vi "BCU参数读取-Auto.vi"(8 "CAN端口":u16(ring), 9 "设备索引号":u16(ring), 10 "CAN卡类型":u32(ring)=21, 11 "Myindex":dbl=1.0) -> (3 "成功":bool)   [LabVIEW 2013] (continued)
                            n1192 = local read "CAN端口"() -> (w1917:u16)
                            n1193 = local write "命令序号"(w1922) -> ()
                            n1194 = stacked-sequence {
                              tunnel: w1923 -> [_ w1931]
                              tunnel: w1922 -> [_ w1930]
                              tunnel: w1921 -> [_ w1929]
                              tunnel: w1920 -> [_ w1928]
                              tunnel: w1919 -> [_ w1927]
                              tunnel: w1918 -> [_ w1926]
                              tunnel: w1917 -> [_ w1925]
                              frame #0 {
                              }
                              frame #1 {
                                n1195 = control-ref of="流控帧"() -> (w1924:refnum<vi>)
                                n1196 = call "多帧发送机制(EV05).vi"("can卡类型"=w1927, "设备索引号"=w1926, "CAN端口"=w1925, "命令"=w1931, "板号"=w1929, "命令序号"=w1930, "输入数据"=w1928, "流控帧"=w1924) -> ()  [unwired: 1 in, 11 out]
                              }
                            }
                          }
                          frame #4 {
                            n1197 = while {
                              tunnel: [w1936] -> w1933
                              tunnel: [w1934] -> w1932
                              i -> [w1939]
                              stop <- w1936 stop-if-true
                              n1198 = local read "强制终止读写标记"() -> (w1935:bool)
                              n1199 = local read "写入超时"() -> (w1934:bool)
                              n1200 = Greater Or Equal?(x=w1939, y=20) -> (x >= y?=w1937:bool)
                              n1201 = Compound Arithmetic op=OR(w1935, w1934, w1937) -> (w1936:bool)
                              n1202 = Wait Until Next ms Multiple(millisecond multiple=u32 100 ("毫秒倍数")) -> ()  [unwired: 1 out]
                            }
                          }
                          frame #5 {
                            n1203 = case shown="假" w1948 {
                              tunnel: w1947 -> [w1959 _]
                              tunnel: [w1954 w1971] -> w1946
                              tunnel: w1945 -> [w1953 _]
                              tunnel: w1944 -> [w1952 w1971]
                              tunnel: [w1951 w1970] -> w1941
                              tunnel: w1943 -> [w1950 _]
                              tunnel: w1942 -> [w1949 w1970]
                              frame False {
                                n1204 = local read "重试次数"() -> (w1958:u8)
                                n1205 = Increment(x=w1958) -> (x+1=w1957:u8)
                                n1206 = local write "重试次数"(w1957) -> ()
                                n1207 = Greater Or Equal?(x=w1957, y=u8 4) -> (x >= y?=w1956:bool)
                                n1208 = case shown="真" w1956 {
                                tunnel: w1959 -> [_ w1964]
                                tunnel: [w1961 w1963] -> w1954
                                tunnel: w1953 -> [w1961 _]
                                tunnel: w1952 -> [_ w1963]
                                tunnel: [w1960 w1962] -> w1951
                                tunnel: w1950 -> [w1960 _]
                                tunnel: w1949 -> [_ w1962]
                                frame False {
                                }
                                frame True {
                                n1209 = control-ref of="结果"() -> (w1966:refnum<vi>)
                                n1210 = Concatenate Strings(w1964, "     读取失败" ("字符串")) -> (w1968:string)
                                n1211 = Build Array(w1968) -> (w1965:string[])
                                n1212 = call "表格编辑.vi"("新元素/子数组"=w1965, "活动单元格:单元格背景色"=u32 16740749, "MCListbox引用句柄"=w1966) -> ()  [unwired: 9 out]
                                }
                                }
                              }
                              frame True {
                              }
                            }
                          }
                          frame #6 {
                            n1213 = And(x=w1973, y=w1975) -> (x .and. y?=w1974:bool)
                            n1214 = case shown="真" w1974 {
                              frame False {
                              }
                              frame True {
                                n1215 = local write "强制终止读写标记"(FALSE ("强制停止")) -> ()
                                n1216 = control-ref of="结果"() -> (w1978:refnum<vi>)
                                n1217 = Concatenate Strings("读取完成" ("字符串")) -> (w1980:string)
                                n1218 = Build Array(w1980) -> (w1977:string[])
                                n1219 = call "表格编辑.vi"("新元素/子数组"=w1977, "活动单元格:单元格背景色"=u32 21937, "MCListbox引用句柄"=w1978) -> ()  [unwired: 9 out]
                              }
                            }
                            n1220 = Wait (ms)(milliseconds to wait=u32 100 ("等待时间（毫秒）")) -> ()  [unwired: 1 out]
                          }
                        }
                      }
                    }
                  }
                  n1221 = local read "强制终止读写标记"() -> (w1745:bool)
                  n1222 = Or(x=w1745, y=w1744) -> (x .or. y?=w1742:bool)
                }
              }
            }
            frame #3 {
              n1223 = case shown="假" FALSE {
                tunnel: w2072 -> [w2073 _]
                frame False {
                  n1224 = case shown="\"主板\", 默认" w2073 {
                    frame "主板", Default {
                      w2074 = "BCURESULT" ("section")
                      n1225 = global read "读配置文件全局.vi" "电池额定实际容量判定"() -> (w2096:bool)
                      n1226 = global read "读配置文件全局.vi" "电池充放电次数判定"() -> (w2085:bool)
                      n1227 = global read "读配置文件全局.vi" "加热控制参数判定"() -> (w2083:bool)
                      n1228 = global read "读配置文件全局.vi" "配置文件版本判定"() -> (w2095:bool)
                      n1229 = global read "读配置文件全局.vi" "充电控制参数判定"() -> (w2089:bool)
                      n1230 = global read "读配置文件全局.vi" "通道电压数判定"() -> (w2101:bool)
                      n1231 = global read "读配置文件全局.vi" "电压起始值判定"() -> (w2100:bool)
                      n1232 = global read "读配置文件全局.vi" "温度起始值判定"() -> (w2098:bool)
                      n1233 = global read "读配置文件全局.vi" "充放电安时判定"() -> (w2087:bool)
                      n1234 = global read "读配置文件全局.vi" "电池包组号判定"() -> (w2086:bool)
                      n1235 = global read "读配置文件全局.vi" "电池信息1判定"() -> (w2088:bool)
                      n1236 = global read "读配置文件全局.vi" "从板个数判定"() -> (w2104:bool)
                      n1237 = global read "读配置文件全局.vi" "产品编号判定"() -> (w2103:bool)
                      n1238 = global read "读配置文件全局.vi" "电压个数判定"() -> (w2102:bool)
                      n1239 = global read "读配置文件全局.vi" "温度个数判定"() -> (w2099:bool)
                      n1240 = global read "读配置文件全局.vi" "保险位置判定"() -> (w2097:bool)
                      n1241 = global read "读配置文件全局.vi" "一级故障判定"() -> (w2092:bool)
                      n1242 = global read "读配置文件全局.vi" "二级故障判定"() -> (w2091:bool)
                      n1243 = global read "读配置文件全局.vi" "三级故障判定"() -> (w2090:bool)
                      n1244 = global read "读配置文件全局.vi" "车牌号判定"() -> (w2094:bool)
                      n1245 = global read "读配置文件全局.vi" "SOH判定"() -> (w2093:bool)
                      n1246 = Build Array(w2104, w2103, w2102, w2101, w2100, w2099, w2098, w2097, w2096, w2095, w2094, w2093, w2092, w2091, w2090, w2089, w2088, w2087, w2086, w2085, w2083) -> (w2084:bool[])
                      n1247 = And Array Elements(Boolean array=w2084) -> (logical AND=w2105:bool)
                      "成功" <- w2105
                      n1248 = case shown="真" w2105 {
                        tunnel: w2084 -> [_ w2126]
                        tunnel: ["PASS" ("section") "FAIL" ("section")] -> w2075
                        frame True {
                          n1249 = control-ref of="结果"() -> (w2122:refnum<vi>)
                          n1250 = Build Array("全部判定成功!!!!!!!!") -> (w2123:string[])
                          n1251 = call "表格编辑.vi"("新元素/子数组"=w2123, "活动单元格:单元格背景色"=u32 6618880, "MCListbox引用句柄"=w2122) -> ()  [unwired: 9 out]
                          n1252 = local write "停止"(TRUE ("停止")) -> ()
                        }
                        frame False {
                          n1253 = stacked-sequence {
                            tunnel: w2126 -> [_ w2131]
                            frame #0 {
                              n1254 = control-ref of="结果"() -> (w2129:refnum<vi>)
                              n1255 = Build Array("全部判定失败!!!!!") -> (w2130:string[])
                              n1256 = call "表格编辑.vi"("新元素/子数组"=w2130, "活动单元格:单元格背景色"=u32 16711680, "MCListbox引用句柄"=w2129) -> ()  [unwired: 9 out]
                            }
                            frame #1 {
                              n1257 = for {
                                tunnel: w2131 -> [w2133] mode=indexing
                                i -> [w2132]
                                n1258 = case shown="17" w2132 {
                                tunnel: w2133 -> [w2134 w2139 w2144 w2149 w2154 w2159 w2164 w2169 w2174 w2179 w2184 w2189 w2194 w2199 w2204 w2209 w2214 w2219 w2224 w2229 w2234 _]
                                frame 0 {
                                n1259 = case shown="假" w2134 {
                                frame False {
                                n1260 = control-ref of="结果"() -> (w2137:refnum<vi>)
                                n1261 = Build Array("从板个数判定失败!") -> (w2138:string[])
                                n1262 = call "表格编辑.vi"("新元素/子数组"=w2138, "活动单元格:单元格背景色"=u32 16711680, "MCListbox引用句柄"=w2137) -> ()  [unwired: 9 out]
                                }
                                frame True {
                                }
                                }
                                }
                                frame 1 {
                                n1263 = case shown="假" w2139 {
                                frame False {
                                n1264 = control-ref of="结果"() -> (w2142:refnum<vi>)
                                n1265 = Build Array("产品编号判定失败!") -> (w2143:string[])
                                n1266 = call "表格编辑.vi"("新元素/子数组"=w2143, "活动单元格:单元格背景色"=u32 16711680, "MCListbox引用句柄"=w2142) -> ()  [unwired: 9 out]
                                }
                                frame True {
                                }
                                }
                                }
                                frame 2 {
                                n1267 = case shown="假" w2144 {
                                frame False {
                                n1268 = control-ref of="结果"() -> (w2147:refnum<vi>)
                                n1269 = Build Array("电压个数判定失败!") -> (w2148:string[])
                                n1270 = call "表格编辑.vi"("新元素/子数组"=w2148, "活动单元格:单元格背景色"=u32 16711680, "MCListbox引用句柄"=w2147) -> ()  [unwired: 9 out]
                                }
                                frame True {
                                }
                                }
                                }
                                frame 3 {
                                n1271 = case shown="假" w2149 {
                                frame False {
                                n1272 = control-ref of="结果"() -> (w2152:refnum<vi>)
                                n1273 = Build Array("通道电压数判定失败!") -> (w2153:string[])
                                n1274 = call "表格编辑.vi"("新元素/子数组"=w2153, "活动单元格:单元格背景色"=u32 16711680, "MCListbox引用句柄"=w2152) -> ()  [unwired: 9 out]
                                }
                                frame True {
                                }
                                }
                                }
                                frame 4 {
                                n1275 = case shown="假" w2154 {
                                frame False {
                                n1276 = control-ref of="结果"() -> (w2157:refnum<vi>)
                                n1277 = Build Array("电压起始值判定失败!") -> (w2158:string[])
                                n1278 = call "表格编辑.vi"("新元素/子数组"=w2158, "活动单元格:单元格背景色"=u32 16711680, "MCListbox引用句柄"=w2157) -> ()  [unwired: 9 out]
                                }
                                frame True {
                                }
                                }
                                }
                                frame 5 {
                                n1279 = case shown="假" w2159 {
                                frame False {
                                n1280 = control-ref of="结果"() -> (w2162:refnum<vi>)
                                n1281 = Build Array("温度个数判定失败!") -> (w2163:string[])
                                n1282 = call "表格编辑.vi"("新元素/子数组"=w2163, "活动单元格:单元格背景色"=u32 16711680, "MCListbox引用句柄"=w2162) -> ()  [unwired: 9 out]
                                }
                                frame True {
                                }
                                }
                                }
                                frame 6 {
                                n1283 = case shown="假" w2164 {
                                frame False {
                                n1284 = control-ref of="结果"() -> (w2167:refnum<vi>)
                                n1285 = Build Array("温度起始值判定失败!") -> (w2168:string[])
                                n1286 = call "表格编辑.vi"("新元素/子数组"=w2168, "活动单元格:单元格背景色"=u32 16711680, "MCListbox引用句柄"=w2167) -> ()  [unwired: 9 out]
                                }
                                frame True {
                                }
                                }
                                }
                                frame 7 {
                                n1287 = case shown="假" w2169 {
                                frame False {
                                n1288 = control-ref of="结果"() -> (w2172:refnum<vi>)
                                n1289 = Build Array("保险位置判定失败!") -> (w2173:string[])
                                n1290 = call "表格编辑.vi"("新元素/子数组"=w2173, "活动单元格:单元格背景色"=u32 16711680, "MCListbox引用句柄"=w2172) -> ()  [unwired: 9 out]
                                }
                                frame True {
                                }
                                }
                                }
                                frame 8 {
                                n1291 = case shown="假" w2174 {
                                frame False {
                                n1292 = control-ref of="结果"() -> (w2177:refnum<vi>)
                                n1293 = Build Array("电池额定实际容量判定失败!") -> (w2178:string[])
                                n1294 = call "表格编辑.vi"("新元素/子数组"=w2178, "活动单元格:单元格背景色"=u32 16711680, "MCListbox引用句柄"=w2177) -> ()  [unwired: 9 out]
                                }
                                frame True {
                                }
                                }
                                }
                                frame 9 {
                                n1295 = case shown="假" w2179 {
                                frame False {
                                n1296 = control-ref of="结果"() -> (w2182:refnum<vi>)
                                n1297 = Build Array("配置文件版本判定失败!") -> (w2183:string[])
                                n1298 = call "表格编辑.vi"("新元素/子数组"=w2183, "活动单元格:单元格背景色"=u32 16711680, "MCListbox引用句柄"=w2182) -> ()  [unwired: 9 out]
                                }
                                frame True {
                                }
                                }
                                }
                                frame 10 {
                                n1299 = case shown="假" w2184 {
                                frame False {
                                n1300 = control-ref of="结果"() -> (w2187:refnum<vi>)
                                n1301 = Build Array("车牌号判定失败!") -> (w2188:string[])
                                n1302 = call "表格编辑.vi"("新元素/子数组"=w2188, "活动单元格:单元格背景色"=u32 16711680, "MCListbox引用句柄"=w2187) -> ()  [unwired: 9 out]
                                }
                                frame True {
                                }
                                }
                                }
                                frame 11 {
                                n1303 = case shown="假" w2189 {
                                frame False {
                                n1304 = control-ref of="结果"() -> (w2192:refnum<vi>)
                                n1305 = Build Array("SOH判定失败!") -> (w2193:string[])
                                n1306 = call "表格编辑.vi"("新元素/子数组"=w2193, "活动单元格:单元格背景色"=u32 16711680, "MCListbox引用句柄"=w2192) -> ()  [unwired: 9 out]
                                }
                                frame True {
                                }
                                }
                                }
                                frame 12 {
                                n1307 = case shown="假" w2194 {
                                frame False {
                                n1308 = control-ref of="结果"() -> (w2197:refnum<vi>)
                                n1309 = Build Array("一级故障阀值判定失败!") -> (w2198:string[])
                                n1310 = call "表格编辑.vi"("新元素/子数组"=w2198, "活动单元格:单元格背景色"=u32 16711680, "MCListbox引用句柄"=w2197) -> ()  [unwired: 9 out]
                                }
                                frame True {
                                }
                                }
                                }
                                frame 13 {
                                n1311 = case shown="假" w2199 {
                                frame False {
                                n1312 = control-ref of="结果"() -> (w2202:refnum<vi>)
                                n1313 = Build Array("二级故障阀值判定失败!") -> (w2203:string[])
                                n1314 = call "表格编辑.vi"("新元素/子数组"=w2203, "活动单元格:单元格背景色"=u32 16711680, "MCListbox引用句柄"=w2202) -> ()  [unwired: 9 out]
                                }
                                frame True {
                                }
                                }
                                }
                                frame 14 {
                                n1315 = case shown="假" w2204 {
                                frame False {
                                n1316 = control-ref of="结果"() -> (w2207:refnum<vi>)
                                n1317 = Build Array("三级故障阀值判定失败!") -> (w2208:string[])
                                n1318 = call "表格编辑.vi"("新元素/子数组"=w2208, "活动单元格:单元格背景色"=u32 16711680, "MCListbox引用句柄"=w2207) -> ()  [unwired: 9 out]
                                }
                                frame True {
                                }
                                }
                                }
                                frame 15 {
                                n1319 = case shown="假" w2209 {
                                frame False {
                                n1320 = control-ref of="结果"() -> (w2212:refnum<vi>)
                                n1321 = Build Array("充电控制参数判定失败!") -> (w2213:string[])
                                n1322 = call "表格编辑.vi"("新元素/子数组"=w2213, "活动单元格:单元格背景色"=u32 16711680, "MCListbox引用句柄"=w2212) -> ()  [unwired: 9 out]
                                }
                                frame True {
                                }
                                }
                                }
                                frame 16 {
                                n1323 = case shown="假" w2214 {
                                frame False {
                                n1324 = control-ref of="结果"() -> (w2217:refnum<vi>)
                                n1325 = Build Array("电池信息1判定失败!") -> (w2218:string[])
                                n1326 = call "表格编辑.vi"("新元素/子数组"=w2218, "活动单元格:单元格背景色"=u32 16711680, "MCListbox引用句柄"=w2217) -> ()  [unwired: 9 out]
                                }
                                frame True {
                                }
                                }
                                }
                                frame 17 {
                                n1327 = case shown="假" w2219 {
                                frame False {
                                n1328 = control-ref of="结果"() -> (w2222:refnum<vi>)
                                n1329 = Build Array("充放电安时判定失败!") -> (w2223:string[])
                                n1330 = call "表格编辑.vi"("新元素/子数组"=w2223, "活动单元格:单元格背景色"=u32 16711680, "MCListbox引用句柄"=w2222) -> ()  [unwired: 9 out]
                                }
                                frame True {
                                }
                                }
                                }
                                frame 18 {
                                n1331 = case shown="假" w2224 {
                                frame False {
                                n1332 = control-ref of="结果"() -> (w2227:refnum<vi>)
                                n1333 = Build Array("电池包组号判定失败!") -> (w2228:string[])
                                n1334 = call "表格编辑.vi"("新元素/子数组"=w2228, "活动单元格:单元格背景色"=u32 16711680, "MCListbox引用句柄"=w2227) -> ()  [unwired: 9 out]
                                }
                                frame True {
                                }
                                }
                                }
                                frame 19 {
                                n1335 = case shown="假" w2229 {
                                frame False {
                                n1336 = control-ref of="结果"() -> (w2232:refnum<vi>)
                                n1337 = Build Array("电池充放电次数判定失败!") -> (w2233:string[])
                                n1338 = call "表格编辑.vi"("新元素/子数组"=w2233, "活动单元格:单元格背景色"=u32 16711680, "MCListbox引用句柄"=w2232) -> ()  [unwired: 9 out]
                                }
                                frame True {
                                }
                                }
                                }
                                frame 20 {
                                n1339 = case shown="假" w2234 {
                                frame False {
                                n1340 = control-ref of="结果"() -> (w2237:refnum<vi>)
                                n1341 = Build Array("加热控制参数判定失败!") -> (w2238:string[])
                                n1342 = call "表格编辑.vi"("新元素/子数组"=w2238, "活动单元格:单元格背景色"=u32 16711680, "MCListbox引用句柄"=w2237) -> ()  [unwired: 9 out]
                                }
                                frame True {
                                }
                                }
                                }
                                frame 99, Default {
                                }
                                }
                              }
                            }
                          }
                          n1343 = local write "停止"(TRUE ("停止")) -> ()
                        }
                      }
                      n1344 = call <vilib>:"Open Config Data.vi"("create file if necessary (T)"=FALSE, "configuration file path"=path "D:/BlueWay/configresult.ini") -> ("error out"=w2079:errorcluster, "refnum"=w2080:T25)  [unwired: 7 in, 1 out]
                      n1345 = call-poly <vilib>:"Write Key.vi"("section"=w2074, "error in (no error)"=w2079, "value"=w2075, "key"=w2074, "refnum"=w2080) -> ("error out"=w2077:errorcluster, "refnum out"=w2078:T25)  [unwired: 4 in, 1 out]
                      n1346 = call <vilib>:"Close Config Data.vi"("error in (no error)"=w2077, "refnum"=w2078) -> ("error out"=w2076:errorcluster)  [unwired: 8 in, 1 out]
                      n1347 = stacked-sequence {
                        seq-local: [w2117] -> [_]
                        tunnel: w2076 -> [w2117]
                        frame #0 {
                          w2106 = u8 0 items=["Normal", "Listen Only"] ("工作方式")
                          w2112 = u8 1 items=["Dual Filter", "Single Filter"] ("滤波方式")
                          n1348 = local read "CAN卡类型"() -> (w2107:u32)
                          n1349 = local read "设备索引号"() -> (w2108:u16)
                          n1350 = local read "CAN端口"() -> (w2109:u16)
                          n1351 = call "CAN_Init-8.6.vi"("CAN卡类型"=w2107, "设备索引号"=w2108, "CAN端口"=w2109, "操作类型"=enum16{"初始化CAN", "关闭CAN"}."初始化CAN", "滤波方式"=w2112, "Accept Code"=u32 0, "簇"=T21 {"打开CAN"=FALSE, "初始化CAN"=TRUE, "开始CAN"=TRUE, "重启"=TRUE, "关闭CAN"=FALSE}, "Mask Code"=u32 4294967295 ("Accept Code"), "工作方式"=w2106, "是否滤波"=FALSE, "滤波选择"=T20 {"fiter_mode"=1, "fiter_endid"=402653184, "fiter_startid"=419430399}) -> ()  [unwired: 3 in, 6 out]
                        }
                      }
                    }
                    frame "从板" {
                      n1352 = global read "读配置文件全局2.vi" "电压起始值判定"() -> (w2247:bool)
                      n1353 = global read "读配置文件全局2.vi" "温度起始值判定"() -> (w2244:bool)
                      n1354 = global read "读配置文件全局2.vi" "加热控制参数判定"() -> (w2239:bool)
                      n1355 = global read "读配置文件全局2.vi" "通道电压判定"() -> (w2246:bool)
                      n1356 = global read "读配置文件全局2.vi" "保险位置判定"() -> (w2245:bool)
                      n1357 = global read "读配置文件全局2.vi" "一级故障判定"() -> (w2242:bool)
                      n1358 = global read "读配置文件全局2.vi" "二级故障判定"() -> (w2241:bool)
                      n1359 = global read "读配置文件全局2.vi" "三级故障判定"() -> (w2240:bool)
                      n1360 = global read "读配置文件全局2.vi" "从板号判定"() -> (w2248:bool)
                      n1361 = Build Array(w2248, w2247, w2246, w2245, w2244, w2242, w2241, w2240, w2239) -> (w2243:bool[])
                      n1362 = And Array Elements(Boolean array=w2243) -> (logical AND=w2249:bool)
                      n1363 = case shown="假" w2249 {
                        tunnel: w2243 -> [_ w2254]
                        frame True {
                          n1364 = control-ref of="结果"() -> (w2252:refnum<vi>)
                          n1365 = Build Array("读取判定成功!!!!!!!!") -> (w2253:string[])
                          n1366 = call "表格编辑.vi"("新元素/子数组"=w2253, "活动单元格:单元格背景色"=u32 6618880, "MCListbox引用句柄"=w2252) -> ()  [unwired: 9 out]
                        }
                        frame False {
                          n1367 = stacked-sequence {
                            tunnel: w2254 -> [_ w2259]
                            frame #0 {
                              n1368 = control-ref of="结果"() -> (w2257:refnum<vi>)
                              n1369 = Build Array("读取判定失败!!!!!") -> (w2258:string[])
                              n1370 = call "表格编辑.vi"("新元素/子数组"=w2258, "活动单元格:单元格背景色"=u32 16711680, "MCListbox引用句柄"=w2257) -> ()  [unwired: 9 out]
                            }
                            frame #1 {
                              n1371 = for {
                                tunnel: w2259 -> [w2260] mode=indexing
                                i -> [w2261]
                                n1372 = case shown="0" w2261 {
                                tunnel: w2260 -> [w2262 w2267 w2272 w2277 w2282 w2287 w2292 w2297 w2302 _]
                                frame 0 {
                                n1373 = case shown="假" w2262 {
                                frame False {
                                n1374 = control-ref of="结果"() -> (w2265:refnum<vi>)
                                n1375 = Build Array("从板号判定失败!") -> (w2266:string[])
                                n1376 = call "表格编辑.vi"("新元素/子数组"=w2266, "活动单元格:单元格背景色"=u32 16711680, "MCListbox引用句柄"=w2265) -> ()  [unwired: 9 out]
                                }
                                frame True {
                                }
                                }
                                }
                                frame 1 {
                                n1377 = case shown="假" w2267 {
                                frame False {
                                n1378 = control-ref of="结果"() -> (w2270:refnum<vi>)
                                n1379 = Build Array("电压起始值判定失败!") -> (w2271:string[])
                                n1380 = call "表格编辑.vi"("新元素/子数组"=w2271, "活动单元格:单元格背景色"=u32 16711680, "MCListbox引用句柄"=w2270) -> ()  [unwired: 9 out]
                                }
                                frame True {
                                }
                                }
                                }
                                frame 2 {
                                n1381 = case shown="假" w2272 {
                                frame False {
                                n1382 = control-ref of="结果"() -> (w2275:refnum<vi>)
                                n1383 = Build Array("通道电压节数判定失败!") -> (w2276:string[])
                                n1384 = call "表格编辑.vi"("新元素/子数组"=w2276, "活动单元格:单元格背景色"=u32 16711680, "MCListbox引用句柄"=w2275) -> ()  [unwired: 9 out]
                                }
                                frame True {
                                }
                                }
                                }
                                frame 3 {
                                n1385 = case shown="假" w2277 {
                                frame False {
                                n1386 = control-ref of="结果"() -> (w2280:refnum<vi>)
                                n1387 = Build Array("保险位置判定失败!") -> (w2281:string[])
                                n1388 = call "表格编辑.vi"("新元素/子数组"=w2281, "活动单元格:单元格背景色"=u32 16711680, "MCListbox引用句柄"=w2280) -> ()  [unwired: 9 out]
                                }
                                frame True {
                                }
                                }
                                }
                                frame 4 {
                                n1389 = case shown="假" w2282 {
                                frame False {
                                n1390 = control-ref of="结果"() -> (w2285:refnum<vi>)
                                n1391 = Build Array("温度起始值判定失败!") -> (w2286:string[])
                                n1392 = call "表格编辑.vi"("新元素/子数组"=w2286, "活动单元格:单元格背景色"=u32 16711680, "MCListbox引用句柄"=w2285) -> ()  [unwired: 9 out]
                                }
                                frame True {
                                }
                                }
                                }
                                frame 5 {
                                n1393 = case shown="假" w2287 {
                                frame False {
                                n1394 = control-ref of="结果"() -> (w2290:refnum<vi>)
                                n1395 = Build Array("一级故障判定失败!") -> (w2291:string[])
                                n1396 = call "表格编辑.vi"("新元素/子数组"=w2291, "活动单元格:单元格背景色"=u32 16711680, "MCListbox引用句柄"=w2290) -> ()  [unwired: 9 out]
                                }
                                frame True {
                                }
                                }
                                }
                                frame 6 {
                                n1397 = case shown="假" w2292 {
                                frame False {
                                n1398 = control-ref of="结果"() -> (w2295:refnum<vi>)
                                n1399 = Build Array("二级故障判定失败!") -> (w2296:string[])
                                n1400 = call "表格编辑.vi"("新元素/子数组"=w2296, "活动单元格:单元格背景色"=u32 16711680, "MCListbox引用句柄"=w2295) -> ()  [unwired: 9 out]
                                }
                                frame True {
                                }
                                }
                                }
                                frame 7 {
                                n1401 = case shown="假" w2297 {
                                frame False {
                                n1402 = control-ref of="结果"() -> (w2300:refnum<vi>)
                                n1403 = Build Array("三级故障判定失败!") -> (w2301:string[])
                                n1404 = call "表格编辑.vi"("新元素/子数组"=w2301, "活动单元格:单元格背景色"=u32 16711680, "MCListbox引用句柄"=w2300) -> ()  [unwired: 9 out]
                                }
                                frame True {
                                }
                                }
                                }
                                frame 8 {
                                n1405 = case shown="假" w2302 {
                                frame False {
                                n1406 = control-ref of="结果"() -> (w2305:refnum<vi>)
                                n1407 = Build Array("加热控制参数判定失败!") -> (w2306:string[])
                                n1408 = call "表格编辑.vi"("新元素/子数组"=w2306, "活动单元格:单元格背景色"=u32 16711680, "MCListbox引用句柄"=w2305) -> ()  [unwired: 9 out]
                                }
                                frame True {
                                }
                                }
                                }
                                frame 99, Default {
                                }
                                }
                              }
                            }
                          }
                        }
                      }
                      n1409 = disable-structure shown="禁用" {
                        frame Disabled {
                          n1410 = global read "读配置文件全局.vi" "SOC判定"() -> ()  [unwired: 1 out]
                        }
                        frame Enabled {
                        }
                      }
                    }
                  }
                }
                frame True {
                }
              }
            }
          }
          n1411 = stacked-sequence {
            tunnel: w1086 -> [_]
            frame #0 {
              n1412 = local write "强制终止读写标记"(FALSE ("强制停止")) -> ()
            }
          }
          "重试次数" <- u8 0 ("重试次数")
        }
        frame "开启均衡" {
          n1413 = local read "从板板号"() -> (w2307:u8)
          n1414 = stacked-sequence {
            tunnel: 133 -> [_ w2333 _ _]
            tunnel: w2307 -> [_ _ _ _]
            frame #0 {
              w2317 = u8 0 items=["Normal", "Listen Only"] ("工作方式")
              w2316 = u8 1 items=["Dual Filter", "Single Filter"] ("滤波方式")
              n1415 = global write "EV05全局变量1.vi" "读取超时"(FALSE ("读取超时")) -> ()
              n1416 = global write "EV05全局变量1.vi" "流控帧 2"(TRUE ("流控帧 2")) -> ()
              n1417 = local write "写?"(TRUE ("写?")) -> ()
              n1418 = local read "设备索引号"() -> (w2312:u16)
              n1419 = local read "CAN卡类型"() -> (w2311:u32)
              n1420 = local read "CAN端口"() -> (w2313:u16)
              n1421 = local write "控制1"(TRUE ("控制1")) -> ()
              n1422 = local write "消除"(TRUE ("消除")) -> ()
              n1423 = global write "EV05全局变量1.vi" "流控帧"(FALSE ("流控帧")) -> ()
              n1424 = call "CAN_Init-8.6.vi"("CAN卡类型"=w2311, "设备索引号"=w2312, "CAN端口"=w2313, "操作类型"=enum16{"初始化CAN", "关闭CAN"}."初始化CAN", "滤波方式"=w2316, "Accept Code"=u32 606601216, "簇"=T21 {"打开CAN"=FALSE, "初始化CAN"=TRUE, "开始CAN"=TRUE, "重启"=FALSE, "关闭CAN"=FALSE}, "Mask Code"=u32 524287 ("Accept Code"), "工作方式"=w2317, "是否滤波"=TRUE, "滤波选择"=T20 {"fiter_mode"=1, "fiter_endid"=75825152, "fiter_startid"=75890687}) -> ()  [unwired: 3 in, 6 out]
              n1425 = Wait Until Next ms Multiple(millisecond multiple=u32 20 ("毫秒倍数")) -> ()  [unwired: 1 out]
            }
            frame #1 {
              n1426 = local write "命令"(w2333) -> ()
              n1427 = call "ID组合.vi"("SA(4)"=0 ("PDU(1)"), "PS(3)"=63 ("PDU(1)"), "PF(2)"=w2333, "PDU(1)"=4) -> ("ID"=w2332:i32)  [unwired: 7 out]
              n1428 = local read "均衡类型选择"() -> (w2329:enum16{"放电均衡", "充电均衡", "充放电均衡"})
              n1429 = local read "设备索引号"() -> (w2338:u16)
              n1430 = local read "CAN卡类型"() -> (w2339:u32)
              n1431 = local read "CAN端口"() -> (w2337:u16)
              n1432 = local write "命令序号"(2) -> ()
              n1433 = Add(x=w2329, y=1) -> (x+y=w2327:i32)
              n1434 = Build Array(2, 2, w2327) -> (w2340:i32[])
              n1435 = call "transmit-8.6.vi"("can卡类型"=w2339, "设备索引号"=w2338, "CAN端口"=w2337, "ID"=w2332, "SendType"=u8 0, "Data"=w2340) -> ()  [unwired: 3 in, 11 out]
            }
            frame #2 {
              n1436 = Wait Until Next ms Multiple(millisecond multiple=u32 1000 ("毫秒倍数")) -> ()  [unwired: 1 out]
            }
            frame #3 {
              w2348 = u8 0 items=["Normal", "Listen Only"] ("工作方式")
              w2349 = u8 1 items=["Dual Filter", "Single Filter"] ("滤波方式")
              n1437 = global write "EV05全局变量1.vi" "流控帧 2"(FALSE ("流控帧 2")) -> ()
              n1438 = local read "CAN卡类型"() -> (w2354:u32)
              n1439 = local read "设备索引号"() -> (w2353:u16)
              n1440 = local read "CAN端口"() -> (w2352:u16)
              n1441 = local write "控制1"(FALSE ("控制1")) -> ()
              n1442 = local write "消除"(FALSE ("消除")) -> ()
              n1443 = call <vilib>:"Unset Busy.vi"() -> ()  [unwired: 2 in, 10 out]
              n1444 = call "CAN_Init-8.6.vi"("CAN卡类型"=w2354, "设备索引号"=w2353, "CAN端口"=w2352, "操作类型"=enum16{"初始化CAN", "关闭CAN"}."初始化CAN", "滤波方式"=w2349, "Accept Code"=u32 3221225472, "簇"=T21 {"打开CAN"=FALSE, "初始化CAN"=TRUE, "开始CAN"=TRUE, "重启"=FALSE, "关闭CAN"=FALSE}, "Mask Code"=u32 1073741823 ("Accept Code"), "工作方式"=w2348, "是否滤波"=TRUE, "滤波选择"=T20 {"fiter_mode"=1, "fiter_endid"=402653184, "fiter_startid"=419430399}) -> ()  [unwired: 3 in, 6 out]
            }
          }
        }
        frame "关闭均衡" {
          n1445 = local read "从板板号"() -> (w2358:u8)
          n1446 = stacked-sequence {
            tunnel: 133 -> [_ w2382 _ _]
            tunnel: w2358 -> [_ _ _ _]
            frame #0 {
              w2368 = u8 0 items=["Normal", "Listen Only"] ("工作方式")
              w2367 = u8 1 items=["Dual Filter", "Single Filter"] ("滤波方式")
              n1447 = global write "EV05全局变量1.vi" "读取超时"(FALSE ("读取超时")) -> ()
              n1448 = global write "EV05全局变量1.vi" "流控帧 2"(TRUE ("流控帧 2")) -> ()
              n1449 = local write "写?"(TRUE ("写?")) -> ()
              n1450 = local read "设备索引号"() -> (w2363:u16)
              n1451 = local read "CAN卡类型"() -> (w2362:u32)
              n1452 = local read "CAN端口"() -> (w2364:u16)
              n1453 = local write "控制1"(TRUE ("控制1")) -> ()
              n1454 = global write "EV05全局变量1.vi" "流控帧"(FALSE ("流控帧")) -> ()
              n1455 = local write "消除"(TRUE ("消除")) -> ()
              n1456 = call "CAN_Init-8.6.vi"("CAN卡类型"=w2362, "设备索引号"=w2363, "CAN端口"=w2364, "操作类型"=enum16{"初始化CAN", "关闭CAN"}."初始化CAN", "滤波方式"=w2367, "Accept Code"=u32 606601216, "簇"=T21 {"打开CAN"=FALSE, "初始化CAN"=TRUE, "开始CAN"=TRUE, "重启"=FALSE, "关闭CAN"=FALSE}, "Mask Code"=u32 524287 ("Accept Code"), "工作方式"=w2368, "是否滤波"=TRUE, "滤波选择"=T20 {"fiter_mode"=1, "fiter_endid"=75825152, "fiter_startid"=75890687}) -> ()  [unwired: 3 in, 6 out]
              n1457 = Wait Until Next ms Multiple(millisecond multiple=u32 20 ("毫秒倍数")) -> ()  [unwired: 1 out]
            }
            frame #1 {
              n1458 = local write "命令"(w2382) -> ()
              n1459 = call "ID组合.vi"("SA(4)"=0 ("PDU(1)"), "PS(3)"=63 ("PDU(1)"), "PF(2)"=w2382, "PDU(1)"=4) -> ("ID"=w2381:i32)  [unwired: 7 out]
              n1460 = local read "均衡类型选择"() -> (w2392:enum16{"放电均衡", "充电均衡", "充放电均衡"})
              n1461 = local write "命令序号"(3) -> ()
              n1462 = local read "设备索引号"() -> (w2387:u16)
              n1463 = local read "CAN卡类型"() -> (w2388:u32)
              n1464 = local read "CAN端口"() -> (w2386:u16)
              n1465 = Add(x=w2392, y=1) -> (x+y=w2390:i32)
              n1466 = Build Array(2, 3, w2390) -> (w2389:i32[])
              n1467 = call "transmit-8.6.vi"("can卡类型"=w2388, "设备索引号"=w2387, "CAN端口"=w2386, "ID"=w2381, "SendType"=u8 0, "Data"=w2389) -> ()  [unwired: 3 in, 11 out]
            }
            frame #2 {
              n1468 = Wait Until Next ms Multiple(millisecond multiple=u32 1000 ("毫秒倍数")) -> ()  [unwired: 1 out]
            }
            frame #3 {
              w2399 = u8 0 items=["Normal", "Listen Only"] ("工作方式")
              w2400 = u8 1 items=["Dual Filter", "Single Filter"] ("滤波方式")
              n1469 = local read "设备索引号"() -> (w2404:u16)
              n1470 = local read "CAN卡类型"() -> (w2405:u32)
              n1471 = global write "EV05全局变量1.vi" "流控帧 2"(FALSE ("流控帧 2")) -> ()
              n1472 = local read "CAN端口"() -> (w2403:u16)
              n1473 = local write "控制1"(FALSE ("控制1")) -> ()
              n1474 = local write "消除"(FALSE ("消除")) -> ()
              n1475 = call "CAN_Init-8.6.vi"("CAN卡类型"=w2405, "设备索引号"=w2404, "CAN端口"=w2403, "操作类型"=enum16{"初始化CAN", "关闭CAN"}."初始化CAN", "滤波方式"=w2400, "Accept Code"=u32 3221225472, "簇"=T21 {"打开CAN"=FALSE, "初始化CAN"=TRUE, "开始CAN"=TRUE, "重启"=FALSE, "关闭CAN"=FALSE}, "Mask Code"=u32 1073741823 ("Accept Code"), "工作方式"=w2399, "是否滤波"=TRUE, "滤波选择"=T20 {"fiter_mode"=1, "fiter_endid"=402653184, "fiter_startid"=419430399}) -> ()  [unwired: 3 in, 6 out]
              n1476 = call <vilib>:"Unset Busy.vi"() -> ()  [unwired: 2 in, 10 out]
            }
          }
        }
        frame "强制均衡" {
          n1477 = local read "从板板号"() -> (w2409:u8)
          n1478 = stacked-sequence {
            tunnel: 133 -> [_ w2440 _ _]
            tunnel: w2409 -> [_ _ _ _]
            frame #0 {
              w2419 = u8 0 items=["Normal", "Listen Only"] ("工作方式")
              w2418 = u8 1 items=["Dual Filter", "Single Filter"] ("滤波方式")
              n1479 = global write "EV05全局变量1.vi" "读取超时"(FALSE ("读取超时")) -> ()
              n1480 = global write "EV05全局变量1.vi" "流控帧 2"(TRUE ("流控帧 2")) -> ()
              n1481 = local write "写?"(TRUE ("写?")) -> ()
              n1482 = local read "设备索引号"() -> (w2414:u16)
              n1483 = local read "CAN卡类型"() -> (w2413:u32)
              n1484 = local write "控制1"(TRUE ("控制1")) -> ()
              n1485 = local read "CAN端口"() -> (w2415:u16)
              n1486 = local write "消除"(TRUE ("消除")) -> ()
              n1487 = global write "EV05全局变量1.vi" "流控帧"(FALSE ("流控帧")) -> ()
              n1488 = call "CAN_Init-8.6.vi"("CAN卡类型"=w2413, "设备索引号"=w2414, "CAN端口"=w2415, "操作类型"=enum16{"初始化CAN", "关闭CAN"}."初始化CAN", "滤波方式"=w2418, "Accept Code"=u32 606601216, "簇"=T21 {"打开CAN"=FALSE, "初始化CAN"=TRUE, "开始CAN"=TRUE, "重启"=FALSE, "关闭CAN"=FALSE}, "Mask Code"=u32 524287 ("Accept Code"), "工作方式"=w2419, "是否滤波"=TRUE, "滤波选择"=T20 {"fiter_mode"=1, "fiter_endid"=75825152, "fiter_startid"=75890687}) -> ()  [unwired: 3 in, 6 out]
              n1489 = Wait Until Next ms Multiple(millisecond multiple=u32 20 ("毫秒倍数")) -> ()  [unwired: 1 out]
            }
            frame #1 {
              n1490 = local read "强制类型"() -> (w2446:enum16{"全通道开启", "单通道开启", "清待均衡时间"})
              n1491 = case shown="\"清待均衡时间\"" w2446 {
                tunnel: [250 252 254] -> w2436
                tunnel: [_ w2465 _] -> w2435
                tunnel: [_ w2464 _] -> w2434
                tunnel: [_ w2455 _] -> w2433
                tunnel: [_ w2448 _] -> w2432
                frame "全通道开启", Default {
                }
                frame "单通道开启" {
                  n1492 = local read "均衡类型选择"() -> (w2463:enum16{"放电均衡", "充电均衡", "充放电均衡"})
                  n1493 = local read "均衡位置"() -> (w2458:u16)
                  n1494 = case shown="\"放电均衡\", 默认" w2463 {
                    tunnel: [0 1] -> w2462
                    frame "放电均衡", Default {
                    }
                    frame "充电均衡" {
                    }
                  }
                  n1495 = Multiply(x="均衡时间", y=6.0) -> (x*y=w2450:dbl)
                  n1496 = Quotient & Remainder(x=w2450, y=256.0) -> (x-y*floor(x/y)=w2448:dbl, floor(x/y)=w2449:dbl)
                  n1497 = call "二进制解析-8.6.vi"("索引"=1, "数值"=w2462) -> ("低位子数组"=w2453:i32[])  [unwired: 1 in, 2 out]
                  n1498 = Quotient & Remainder(x=w2458, y=256.0) -> (x-y*floor(x/y)=w2464:dbl, floor(x/y)=w2465:dbl)
                  n1499 = call "二进制解析-8.6.vi"("索引"=8, "数值"=w2449) -> ("低位子数组"=w2454:i32[])  [unwired: 1 in, 2 out]
                  n1500 = Replace Array Subset(array=w2454, new element=w2453, index=0 ("索引")) -> (w2451:i32[])
                  n1501 = call "数值二进制转十进制-8.6.vi"("子数组"=w2451) -> ("十进制数值"=w2455:i32)  [unwired: 4 in]
                }
                frame "清待均衡时间" {
                }
              }
              n1502 = local write "命令"(w2440) -> ()
              n1503 = call "ID组合.vi"("SA(4)"=0 ("PDU(1)"), "PS(3)"=63 ("PDU(1)"), "PF(2)"=w2440, "PDU(1)"=4) -> ("ID"=w2439:i32)  [unwired: 7 out]
              n1504 = local read "设备索引号"() -> (w2443:u16)
              n1505 = local read "CAN卡类型"() -> (w2444:u32)
              n1506 = local read "CAN端口"() -> (w2442:u16)
              n1507 = local write "命令序号"(w2436) -> ()
              n1508 = Build Array(6, 4, w2436, w2435, w2434, w2433, w2432) -> (w2445:dbl[])
              n1509 = call "transmit-8.6.vi"("can卡类型"=w2444, "设备索引号"=w2443, "CAN端口"=w2442, "ID"=w2439, "SendType"=u8 0, "Data"=w2445) -> ()  [unwired: 3 in, 11 out]
            }
            frame #2 {
              n1510 = Wait Until Next ms Multiple(millisecond multiple=u32 1000 ("毫秒倍数")) -> ()  [unwired: 1 out]
            }
            frame #3 {
              w2479 = u8 0 items=["Normal", "Listen Only"] ("工作方式")
              w2478 = u8 1 items=["Dual Filter", "Single Filter"] ("滤波方式")
              n1511 = global write "EV05全局变量1.vi" "流控帧 2"(FALSE ("流控帧 2")) -> ()
              n1512 = local write "控制1"(FALSE ("控制1")) -> ()
              n1513 = local read "设备索引号"() -> (w2474:u16)
              n1514 = local read "CAN卡类型"() -> (w2473:u32)
              n1515 = local write "消除"(FALSE ("消除")) -> ()
              n1516 = local read "CAN端口"() -> (w2475:u16)
              n1517 = call <vilib>:"Unset Busy.vi"() -> ()  [unwired: 2 in, 10 out]
              n1518 = call "CAN_Init-8.6.vi"("CAN卡类型"=w2473, "设备索引号"=w2474, "CAN端口"=w2475, "操作类型"=enum16{"初始化CAN", "关闭CAN"}."初始化CAN", "滤波方式"=w2478, "Accept Code"=u32 3221225472, "簇"=T21 {"打开CAN"=FALSE, "初始化CAN"=TRUE, "开始CAN"=TRUE, "重启"=FALSE, "关闭CAN"=FALSE}, "Mask Code"=u32 1073741823 ("Accept Code"), "工作方式"=w2479, "是否滤波"=TRUE, "滤波选择"=T20 {"fiter_mode"=1, "fiter_endid"=402653184, "fiter_startid"=419430399}) -> ()  [unwired: 3 in, 6 out]
            }
          }
        }
        frame "项目软件版本读取" {
          n1519 = stacked-sequence {
            seq-local: [_ w2500 _] -> [_ _ w2507]
            frame #0 {
              n1520 = local read "设备索引号"() -> (w2487:u16)
              n1521 = local read "CAN卡类型"() -> (w2488:u32)
              n1522 = local read "CAN端口"() -> (w2486:u16)
              n1523 = stacked-sequence {
                tunnel: w2488 -> [w2491 w2499]
                tunnel: w2487 -> [w2490 w2498]
                tunnel: w2486 -> [w2489 w2497]
                frame #0 {
                  n1524 = dll-call lib="PTH1abs FBluewave New EnergySVN_WorkAutoTest_TestStandtrunkAutoTest_TestStandDriverZlgCanBHN01è¯»ååæ°data\nkerneldlls\nusbcan.dll" fn="VCI_ClearBuffer"("DeviceType"=w2491, "DeviceInd"=w2490, "CANInd"=w2489) -> (error out=w2492:errorcluster)  [unwired: 4 in, 4 out]
                  n1525 = call <vilib>:"Clear Errors.vi"("error in (no error)"=w2492) -> ()  [unwired: 6 in, 1 out]
                }
                frame #1 {
                  w2496 = u8 137 ("命令")
                  w2495 = u32 1 ("命令序号")
                  n1526 = local read "从板板号"() -> (w2493:u8)
                  n1527 = local write "命令"(w2496) -> ()
                  n1528 = call "多帧发送机制(EV05).vi"("can卡类型"=w2499, "设备索引号"=w2498, "CAN端口"=w2497, "命令"=w2496, "板号"=w2493, "命令序号"=w2495, "输入数据"=dbl[] [0.0]) -> ()  [unwired: 2 in, 11 out]
                  n1529 = local write "命令序号"(w2495) -> ()
                }
              }
            }
            frame #1 {
              n1530 = while {
                tunnel: [w2501] -> w2500
                i -> [w2506]
                stop <- w2503 stop-if-true
                n1531 = global read "EV05全局变量1.vi" "写入超时"() -> (w2501:bool)
                n1532 = Greater Or Equal?(x=w2506, y=25) -> (x >= y?=w2504:bool)
                n1533 = Or(x=w2501, y=w2504) -> (x .or. y?=w2503:bool)
                n1534 = Wait Until Next ms Multiple(millisecond multiple=u32 100 ("毫秒倍数")) -> ()  [unwired: 1 out]
              }
            }
            frame #2 {
              n1535 = case shown="假" w2507 {
                frame False {
                  n1536 = control-ref of="结果"() -> (w2509:refnum<vi>)
                  n1537 = Concatenate Strings("项目软件版本" ("字符串"), "     读取失败" ("字符串")) -> (w2512:string)
                  n1538 = Build Array(w2512) -> (w2511:string[])
                  n1539 = call "表格编辑(版本读取).vi"("新元素/子数组"=w2511, "活动单元格:单元格背景色"=u32 16740749, "MCListbox引用句柄"=w2509) -> ()  [unwired: 9 out]
                }
                frame True {
                }
              }
              n1540 = call <vilib>:"Unset Busy.vi"() -> ()  [unwired: 2 in, 10 out]
            }
          }
        }
        frame "读取故障状态" {
          n1541 = stacked-sequence {
            seq-local: [_ w2538 _] -> [_ _ w2545]
            frame #0 {
              n1542 = local read "设备索引号"() -> (w2515:u16)
              n1543 = local read "CAN卡类型"() -> (w2516:u32)
              n1544 = local read "CAN端口"() -> (w2514:u16)
              n1545 = stacked-sequence {
                tunnel: w2516 -> [w2519 w2528]
                tunnel: w2515 -> [w2518 w2527]
                tunnel: w2514 -> [w2517 w2526]
                frame #0 {
                  n1546 = dll-call lib="PTH1abs FBluewave New EnergySVN_WorkAutoTest_TestStandtrunkAutoTest_TestStandDriverZlgCanBHN01è¯»ååæ°data\nkerneldlls\nusbcan.dll" fn="VCI_ClearBuffer"("DeviceType"=w2519, "DeviceInd"=w2518, "CANInd"=w2517) -> (error out=w2520:errorcluster)  [unwired: 4 in, 4 out]
                  n1547 = call <vilib>:"Clear Errors.vi"("error in (no error)"=w2520) -> ()  [unwired: 6 in, 1 out]
                }
                frame #1 {
                  n1548 = local read "从板板号 2"() -> (w2521:u8)
                  n1549 = case shown="1..30" w2521 {
                    tunnel: [u8 133 ("命令") u8 4 ("命令")] -> w2525
                    frame 0, Default {
                    }
                    frame 1..30 {
                    }
                  }
                  n1550 = local read "状态选择"() -> (w2523:T18)
                  n1551 = local write "命令"(w2525) -> ()
                  n1552 = case shown="\"预充电故障,继电器驱动故障\"" w2523 {
                    tunnel: [1 2 3 4 5 6 7] -> w2522
                    frame "电压,内总电压,外总电压,温度,电流,绝缘,系统时钟,充电均衡,放电均衡", Default {
                    }
                    frame "CPU,CPU内部EE存储器,CPU内部FLASH,内部EE存储器,45db存储器" {
                    }
                    frame "CAN检测故障" {
                    }
                    frame "软件故障" {
                    }
                    frame "RS485,RS232检测故障" {
                    }
                    frame "DI,DO,AI,AO检测故障" {
                    }
                    frame "预充电故障,继电器驱动故障" {
                    }
                  }
                  n1553 = call "多帧发送机制(EV05).vi"("can卡类型"=w2528, "设备索引号"=w2527, "CAN端口"=w2526, "命令"=w2525, "板号"=w2521, "命令序号"=w2522, "输入数据"=dbl[] [0.0]) -> ()  [unwired: 2 in, 11 out]
                  n1554 = local write "命令序号"(w2522) -> ()
                }
              }
            }
            frame #1 {
              n1555 = while {
                tunnel: [w2539] -> w2538
                i -> [w2544]
                stop <- w2541 stop-if-true
                n1556 = global read "EV05全局变量1.vi" "写入超时"() -> (w2539:bool)
                n1557 = Greater Or Equal?(x=w2544, y=25) -> (x >= y?=w2542:bool)
                n1558 = Or(x=w2539, y=w2542) -> (x .or. y?=w2541:bool)
                n1559 = Wait Until Next ms Multiple(millisecond multiple=u32 100 ("毫秒倍数")) -> ()  [unwired: 1 out]
              }
            }
            frame #2 {
              n1560 = case shown="真" w2545 {
                frame False {
                  n1561 = Concatenate Strings("故障信息" ("字符串"), "     读取失败" ("字符串")) -> (w2547:string)
                  n1562 = One Button Dialog(message=w2547, button name ("OK")="确定" ("按钮名称（“确定”）")) -> ()  [unwired: 1 out]
                }
                frame True {
                  n1563 = One Button Dialog(message="故障信息读取完成" ("字符串"), button name ("OK")="确定" ("按钮名称（“确定”）")) -> ()  [unwired: 1 out]
                }
              }
              n1564 = call <vilib>:"Unset Busy.vi"() -> ()  [unwired: 2 in, 10 out]
            }
          }
        }
        frame "平台软件版本读取" {
          n1565 = stacked-sequence {
            seq-local: [_ w2567 _] -> [_ _ w2574]
            frame #0 {
              n1566 = local read "设备索引号"() -> (w2554:u16)
              n1567 = local read "CAN卡类型"() -> (w2555:u32)
              n1568 = local read "CAN端口"() -> (w2553:u16)
              n1569 = stacked-sequence {
                tunnel: w2555 -> [w2558 w2566]
                tunnel: w2554 -> [w2557 w2565]
                tunnel: w2553 -> [w2556 w2564]
                tunnel: u8 137 ("命令") -> [_ w2563]
                frame #0 {
                  n1570 = dll-call lib="PTH1abs FBluewave New EnergySVN_WorkAutoTest_TestStandtrunkAutoTest_TestStandDriverZlgCanBHN01è¯»ååæ°data\nkerneldlls\nusbcan.dll" fn="VCI_ClearBuffer"("DeviceType"=w2558, "DeviceInd"=w2557, "CANInd"=w2556) -> (error out=w2559:errorcluster)  [unwired: 4 in, 4 out]
                  n1571 = call <vilib>:"Clear Errors.vi"("error in (no error)"=w2559) -> ()  [unwired: 6 in, 1 out]
                }
                frame #1 {
                  w2562 = u32 2 ("命令序号")
                  n1572 = local read "从板板号"() -> (w2560:u8)
                  n1573 = local write "命令"(w2563) -> ()
                  n1574 = call "多帧发送机制(EV05).vi"("can卡类型"=w2566, "设备索引号"=w2565, "CAN端口"=w2564, "命令"=w2563, "板号"=w2560, "命令序号"=w2562, "输入数据"=dbl[] [0.0]) -> ()  [unwired: 2 in, 11 out]
                  n1575 = local write "命令序号"(w2562) -> ()
                }
              }
            }
            frame #1 {
              n1576 = while {
                tunnel: [w2568] -> w2567
                i -> [w2573]
                stop <- w2570 stop-if-true
                n1577 = global read "EV05全局变量1.vi" "写入超时"() -> (w2568:bool)
                n1578 = Greater Or Equal?(x=w2573, y=25) -> (x >= y?=w2571:bool)
                n1579 = Or(x=w2568, y=w2571) -> (x .or. y?=w2570:bool)
                n1580 = Wait Until Next ms Multiple(millisecond multiple=u32 100 ("毫秒倍数")) -> ()  [unwired: 1 out]
              }
            }
            frame #2 {
              n1581 = case shown="假" w2574 {
                frame False {
                  n1582 = control-ref of="结果"() -> (w2577:refnum<vi>)
                  n1583 = Concatenate Strings("平台软件版本" ("字符串"), "     读取失败" ("字符串")) -> (w2579:string)
                  n1584 = Build Array(w2579) -> (w2576:string[])
                  n1585 = call "表格编辑(版本读取).vi"("新元素/子数组"=w2576, "活动单元格:单元格背景色"=u32 16740749, "MCListbox引用句柄"=w2577) -> ()  [unwired: 9 out]
                }
                frame True {
                }
              }
